vi "MRB_open.vi"(7 "Serial Settings:Baud Rate":u32(ring)=9600 items=["9.6KHz"=9600, "19.2KHz"=19200], 8 "err_in":errorcluster, 11 "thcd_visa":refnum<visa-resource-name>="COM39") -> (0 "err_out":errorcluster, 3 "thcd_visa":refnum<visa-resource-name>, 4 "status":bool)   [LabVIEW 2019]
uses:
  <vilib>/Instr/_visa.llb/VISA Flush IO Buffer Mask.ctl
panel:
  in  "Mask":T1=64 items=["Flush Receive Buffer"=16, "Write Transmit Buffer to Device"=32, "Flush Receive Buffer (No I/O)"=64, "Flush Transmit Buffer"=128]
  in  "Serial Settings:End Mode for Writes":u16(ring)=2 items=["None", "Last Bit", "TermChar", "Break"]
  in  "Serial Settings:End Mode for Reads":u16(ring)=2 items=["None", "Last Bit", "TermChar"]
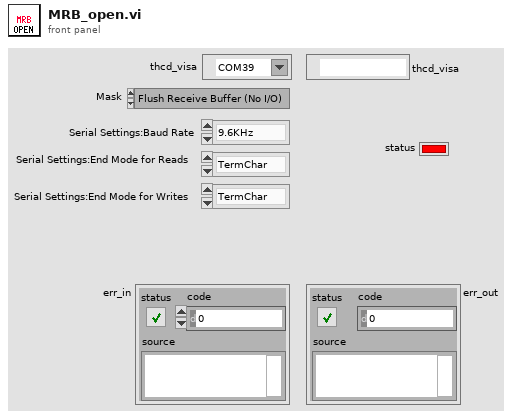
[diagram p1: front panel]
types:
  T1 = typedef "VISA Flush IO Buffer Mask.ctl" = u16
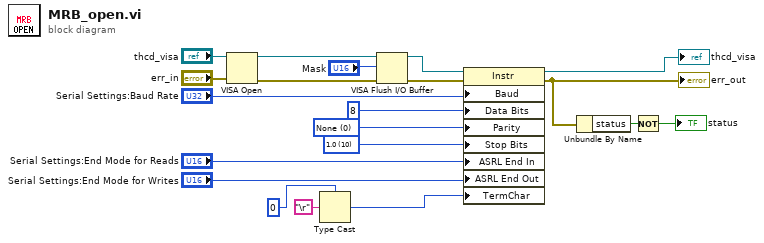
[diagram p0: block diagram]
diagram:
  w17 = u16 10 items=["1.0"=10, "1.5"=15, "2.0"=20] ("Serial Settings:Stop Bits")
  w18 = u16 0 items=["None", "Odd", "Even", "Mark", "Space"] ("Serial Settings:Parity")
  n1 = VISA Open(error in (no error)="err_in", VISA resource name="thcd_visa") -> (VISA resource name=w10:refnum<visa-resource-name>, error out=w9:errorcluster)  [unwired: 3 in]
  n2 = Type Cast(type=u8 0, x="\r") -> (*(type *) &x=w12:u8)
  n3 = VISA Flush I/O Buffer(VISA resource name=w10, mask (16)="Mask", error in (no error)=w9) -> (VISA resource name out=w7:refnum<visa-resource-name>, error out=w8:errorcluster)
  n4 = property class="Instr"(reference=w7, error in=w8, "Baud"="Serial Settings:Baud Rate", "Data Bits"=u16 8 ("Serial Settings:Data Bits"), "Parity"=w18, "Stop Bits"=w17, "ASRL End In"="Serial Settings:End Mode for Reads", "ASRL End Out"="Serial Settings:End Mode for Writes", "TermChar"=w12) -> (reference out=→"thcd_visa":refnum<visa-resource-name>, error out=w3:errorcluster)
  "err_out" <- w3
  n5 = Unbundle By Name(w3) -> ("status"=w2:bool)
  n6 = Not(x=w2) -> (.not. x?=→"status":bool)
